vi "Configure Trigger.vi"(5 "Enable Trigger Delay (T: Enable)":bool=TRUE, 6 "Trigger Delay Time (6E-6 s)":dbl=6e-06, 7 "Video Trigger Level (0)":dbl, 8 "error in (no error)":errorcluster, 9 "Trigger Source (0: Immediate)":i32(ring) items=["Immediate", "Video", "External"], 10 "External Trigger Slope (0: Positive)":i32(ring) items=["Positive", "Negative"], 11 "VISA resource name":refnum<visa-resource-name>) -> (0 "error out":errorcluster, 3 "VISA resource name out":refnum<visa-resource-name>)   [LabVIEW 2022 SP3, in "Agilent N934X Series.lvlib"]
doc: "Configures the trigger settings on the spectrum analyzer."
uses:
  <instrlib>/Agilent N934X Series/Agilent N934X Series.lvlib
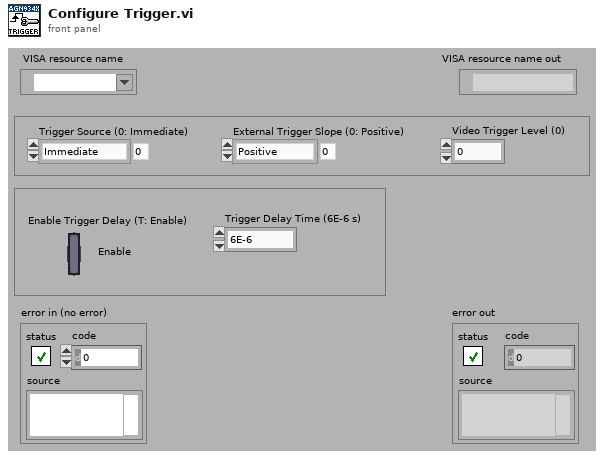
[diagram p1: front panel]
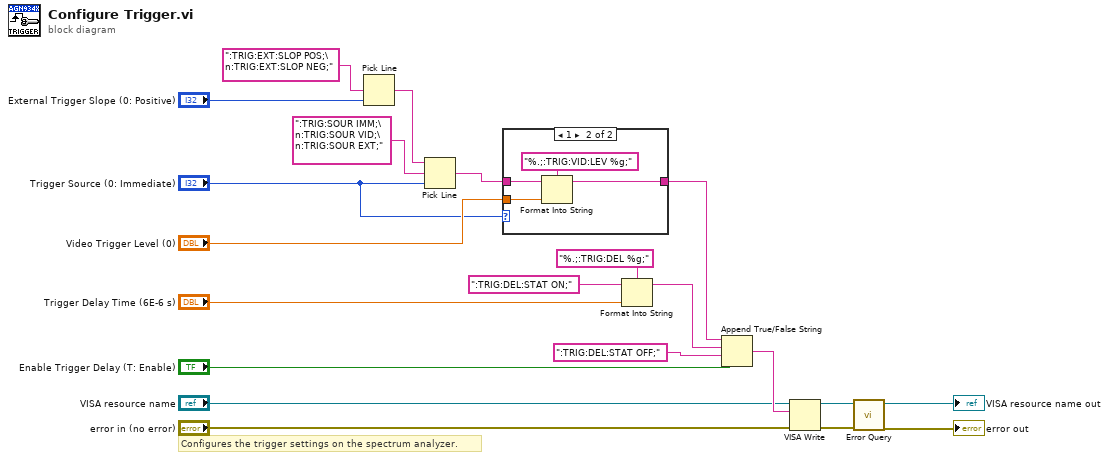
[diagram p0: block diagram]
diagram:
  # "Configures the trigger settings on the spectrum analyzer."
  n1 = Pick Line(multi-line string=":TRIG:EXT:SLOP POS;\n:TRIG:EXT:SLOP NEG;", line index="External Trigger Slope (0: Positive)") -> (output string=w18:string)  [unwired: 1 in]
  n2 = Pick Line(string ("")=w18, multi-line string=":TRIG:SOUR IMM;\n:TRIG:SOUR VID;\n:TRIG:SOUR EXT;", line index="Trigger Source (0: Immediate)") -> (output string=w4:string)
  n3 = case shown="1" "Trigger Source (0: Immediate)" {
    tunnel: w4 -> [w22 w25]
    tunnel: "Video Trigger Level (0)" -> [_ w24]
    tunnel: [w22 w23] -> w1
    frame 0, 2, Default {
    }
    frame 1 {
      n4 = Format Into String(format string="%.;:TRIG:VID:LEV %g;", initial string=w25, w24) -> (resulting string=w23:string)  [unwired: 1 in, 1 out]
    }
  }
  n5 = Format Into String(format string="%.;:TRIG:DEL %g;", initial string=":TRIG:DEL:STAT ON;", "Trigger Delay Time (6E-6 s)") -> (resulting string=w2:string)  [unwired: 1 in, 1 out]
  n6 = Append True/False String(1:"Enable Trigger Delay (T: Enable)", 2:":TRIG:DEL:STAT OFF;", 3:w2, 4:w1) -> (0:w13:string)
  n7 = VISA Write(VISA resource name="VISA resource name", write buffer=w13, error in (no error)="error in (no error)") -> (VISA resource name out=w10:refnum<visa-resource-name>, error out=w9:errorcluster)  [unwired: 1 out]
  n8 = call <instrlib>:"Error Query.vi"("error in (no error)"=w9, "VISA resource name"=w10) -> ("error out"=→"error out":errorcluster, "VISA resource name out"=→"VISA resource name out":refnum<visa-resource-name>)  [unwired: 6 in, 2 out]
